vi "LSCI332 GetZoneInfo.vi"(6 "error in (no error)":errorcluster, 7 "Zone":u32=1 min=1 max=10 step=1, 9 "Boucle(1)":u32(ring) caption="Boucle" items=["Boucle 1", "Boucle 2"], 10 "VISA Rsrc":refnum<visa-resource-name>="GPIB0::12::INSTR") -> (0 "error out":errorcluster, 3 "Paramètres":T1={"TempFin"=400.0, "P"=1000.0, "I"=0.0, "D"=0, "ManualOutput(%)"=0.0, "Range"=5} {"D" max=1000 step=1; "I" min=0.0 max=1000.0 step=0.1 format="%#.1f"; "Range" max=5 step=1; "ManualOutput(%)" min=-100.0 max=100.0 step=0.01 format="%#.2g"; "P" min=0.0 max=1000.0 step=0.1 format="%#.1f"; "TempFin" min=0.0 max=400.0 step=0.001 format="%#.3g"})   [LabVIEW 2019]
doc: "Ce VI envoie la commande Zone? au contrôlleur, ce qui retourne les paramètres de la zone spécifiée."
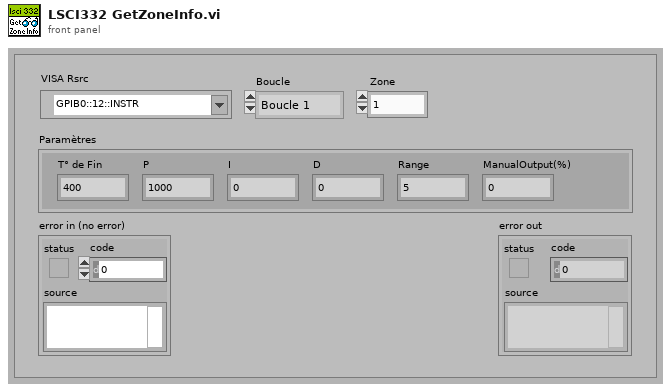
[diagram p1: front panel]
types:
  T1 = cluster{"TempFin":dbl, "P":dbl, "I":dbl, "D":u32, "ManualOutput(%)":dbl, "Range":u32}
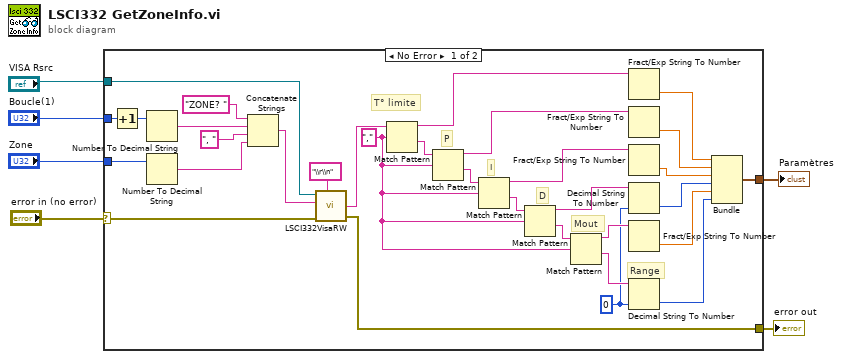
[diagram p0: block diagram]
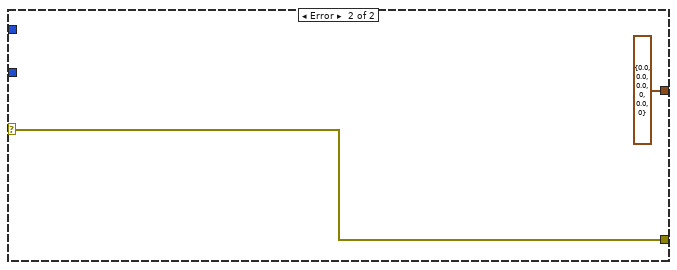
[diagram p2: hidden frame]
diagram:
  n1 = case shown="No Error" "error in (no error)" {
    selector: "error in (no error)" -> [w36 w40]
    tunnel: "VISA Rsrc" -> [w37 _]
    tunnel: "Boucle(1)" -> [w33 _]
    tunnel: "Zone" -> [w34 _]
    tunnel: [w35 w40] -> w3
    tunnel: [w8 cluster{dbl, dbl, dbl, u32, dbl, u32} {0.0, 0.0, 0.0, 0, 0.0, 0}] -> w1
    frame No Error {
      w7 = u32 0 ("default (0 I32)")
      w24 = "," ("regular expression")
      # "Range"
      # "Mout"
      # "D"
      # "I"
      # "P"
      # "T° limite"
      n2 = Increment(x=w33) -> (x+1=w32:u32)
      n3 = Number To Decimal String(number=w32) -> (decimal integer string=w30:string)  [unwired: 1 in]
      n4 = Number To Decimal String(number=w34) -> (decimal integer string=w28:string)  [unwired: 1 in]
      n5 = Concatenate Strings("ZONE? " ("string"), w30, ", " ("string"), w28) -> (w27:string)
      n6 = call <userlib>:"LSCI332VisaRW.vi"("error in (no error)"=w36, "EOS (Aucun)"="\\r\\n", "ChaineCom"=w27, "VISA Rsrc"=w37) -> ("error out"=w35:errorcluster, "ChaineRep"=w26:string)  [unwired: 3 in, 2 out]
      n7 = Match Pattern(string=w26, regular expression=w24) -> (before substring=w20:string, after substring=w25:string)  [unwired: 1 in, 2 out]
      n8 = Match Pattern(string=w25, regular expression=w24) -> (before substring=w19:string, after substring=w23:string)  [unwired: 1 in, 2 out]
      n9 = Match Pattern(string=w23, regular expression=w24) -> (before substring=w18:string, after substring=w22:string)  [unwired: 1 in, 2 out]
      n10 = Match Pattern(string=w22, regular expression=w24) -> (before substring=w17:string, after substring=w21:string)  [unwired: 1 in, 2 out]
      n11 = Match Pattern(string=w21, regular expression=w24) -> (before substring=w15:string, after substring=w16:string)  [unwired: 1 in, 2 out]
      n12 = Fract/Exp String To Number(string=w20) -> (number=w14:dbl)  [unwired: 3 in, 1 out]
      n13 = Fract/Exp String To Number(string=w19) -> (number=w13:dbl)  [unwired: 3 in, 1 out]
      n14 = Fract/Exp String To Number(string=w18) -> (number=w12:dbl)  [unwired: 3 in, 1 out]
      n15 = Decimal String To Number(string=w17, default (0L)=w7) -> (number=w11:u32)  [unwired: 1 in, 1 out]
      n16 = Fract/Exp String To Number(string=w15) -> (number=w10:dbl)  [unwired: 3 in, 1 out]
      n17 = Decimal String To Number(string=w16, default (0L)=w7) -> (number=w9:u32)  [unwired: 1 in, 1 out]
      n18 = Bundle(w14, w13, w12, w11, w10, w9) -> (w8:cluster{dbl, dbl, dbl, u32, dbl, u32})  [unwired: 1 in]
    }
    frame Error {
    }
  }
  "error out" <- w3
  "Paramètres" <- w1
